vi "Timer FGV.vi"(7 "Action":T1, 8 "error in (no error)":errorcluster) -> (0 "error out":errorcluster, 3 "Elapsed Time":dbl)   [LabVIEW 2015]
uses:
  Timer Actions.ctl
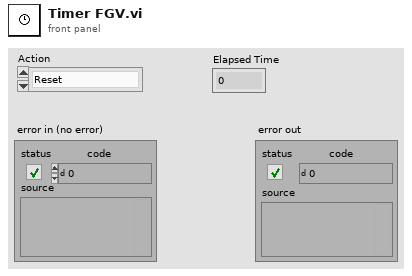
[diagram p1: front panel]
types:
  T1 = typedef "Timer Actions.ctl" = enum16{"Reset", "Get"}
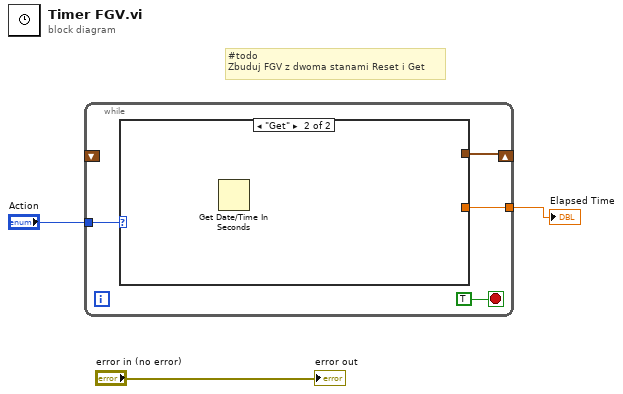
[diagram p0: block diagram]
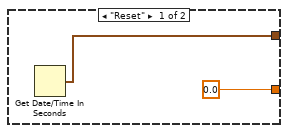
[diagram p2: hidden frame]
diagram:
  # "#todo \nZbuduj FGV z dwoma stanami Reset i Get"
  n1 = while {
    shift-right: [w5] -> _
    shift-left: _ -> [_]
    tunnel: "Action" -> [w6]
    tunnel: [w4] -> w1
    stop <- TRUE stop-if-true
    n2 = case shown="\"Get\"" w6 {
      tunnel: [w9 _] -> w5
      tunnel: [0.0 _] -> w4
      frame "Reset" {
        n3 = Get Date/Time In Seconds() -> (seconds since 1Jan1904=w9:timestamp)
      }
      frame "Get" {
        n4 = Get Date/Time In Seconds() -> ()  [unwired: 1 out]
      }
    }
  }
  "Elapsed Time" <- w1
  "error out" <- "error in (no error)"
